vi "Master Save.vi"(7 "#scans":u32, 8 "Current Scan #":u32, 10 "Data Store":T1, 11 "File IO in":refnum<class "File IO.lvclass">) -> (0 "error out":errorcluster, 3 "File IO out":refnum<class "File IO.lvclass">)   [LabVIEW 2012, in "File IO.lvclass"]
uses:
  File IO.lvclass
  Instruments/Utility Classes/Readable/Data Store.ctl
  Instruments/Utility Classes/Readable/Data Point.ctl
  Instruments/Utility Classes/Readable/Time.ctl
  Instruments/Utility Classes/Readable/X.ctl
  File IO.lvclass/File IO.ctl
  <vilib>/Utility/file.llb/Write To Spreadsheet File (DBL).vi
  Data File Header Constants.vi
  Instruments/Utility Classes/Readable/Readable.lvclass
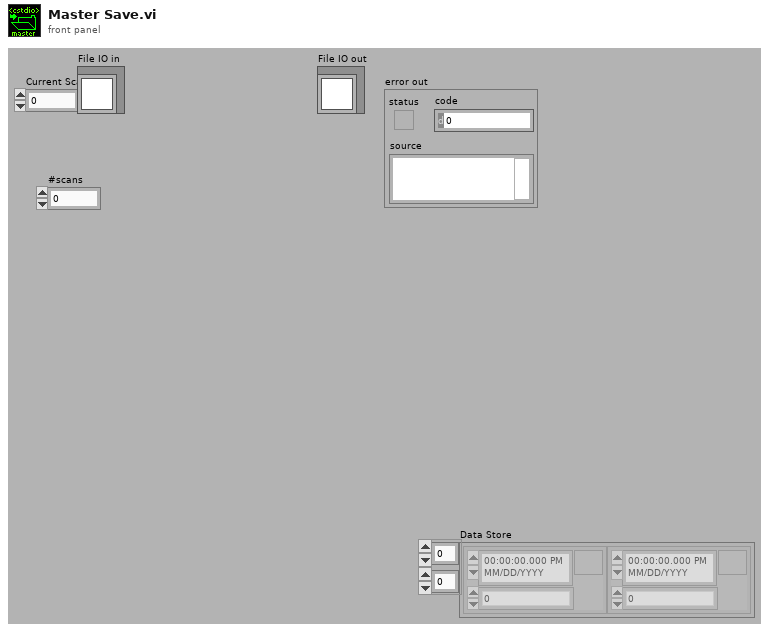
[diagram p1: front panel]
types:
  T1 = typedef "Readable.lvclass/Data Store.ctl" = T2[][]
  T2 = typedef "Readable.lvclass/Data Point.ctl" = cluster{"t":T3, "x":T4}
  T3 = typedef "Readable.lvclass/Time.ctl" = timestamp
  T4 = typedef "Readable.lvclass/X.ctl" = dbl
  T5 = enum16{"open", "replace", "create", "open or create", "replace or create", "replace or create with confirmation"}
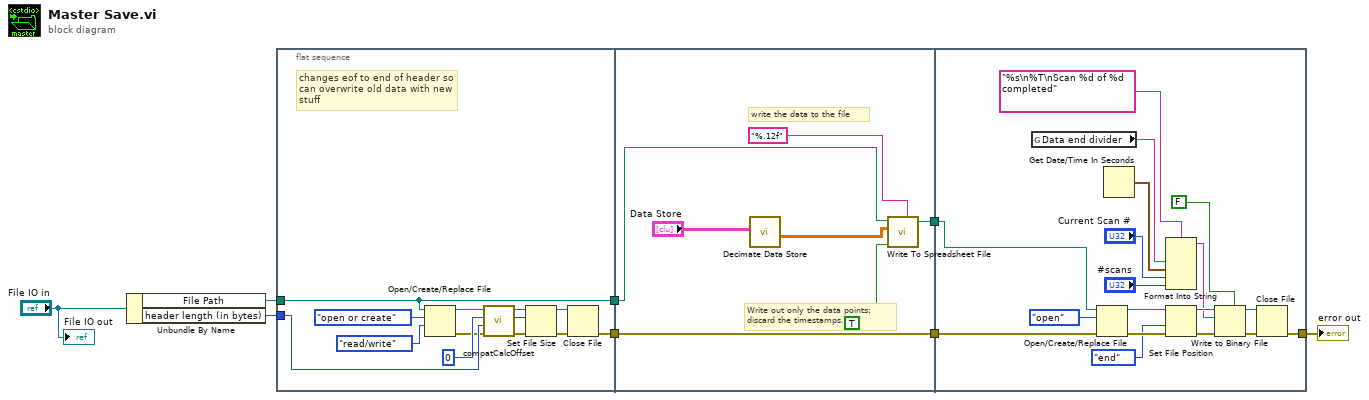
[diagram p0: block diagram]
diagram:
  n1 = Unbundle By Name("File IO in") -> ("File Path"=w7:path, "header length (in bytes)"=w4:u64)
  n2 = flat-sequence {
    tunnel: w7 -> [w13]
    tunnel: [w13] -> w6
    tunnel: w4 -> [w12]
    tunnel: [w9] -> w2
    tunnel: w6 -> [w25]
    tunnel: [w24] -> w5
    tunnel: [w26] -> w3
    tunnel: w2 -> [w26]
    tunnel: w5 -> [w33]
    tunnel: w3 -> [w32]
    tunnel: [w30] -> w1
    frame #0 {
      # "changes eof to end of header so\ncan overwrite old data with new\nstuff"
      n3 = Open/Create/Replace File(file path (use dialog)=w13, operation (0:open)=T5."open or create", access (0:read/write)=enum16{"read/write", "read-only", "write-only"}."read/write") -> (refnum out=w14:refnum<file>, error out=w11:errorcluster)  [unwired: 1 in, 3 out]
      n4 = call <vilib>:"compatCalcOffset.vi"("error in"=w11, "pos offset (0)"=w12, "pos mode (0:1)"=u16 0, "refnum"=w14) -> ("error out"=w20:errorcluster, "offset"=w19:i32, "dup refnum"=w18:refnum<file>)  [unwired: 5 out]
      n5 = Set File Size(4:w20, 6:w19, 7:w18) -> (0:w10:errorcluster, 3:w17:refnum<file>)
      n6 = Close File(refnum=w17, error in=w10) -> (error out=w9:errorcluster)  [unwired: 1 out]
    }
    frame #1 {
      # "Write out only the data points;\ndiscard the timestamps."
      # "write the data to the file"
      n7 = call "Decimate Data Store.vi"("Data Store"="Data Store") -> ("Data Points"=w22:T4[][])  [unwired: 9 in, 1 out]
      n8 = call-poly <vilib>:"Write To Spreadsheet File.vi"("format (%.3f)"="%.12f", "append to file? (new file:F)"=TRUE, "2D data"=w22, "file path (dialog if empty)"=w25) -> ("new file path (Not A Path if cancelled)"=w24:path)  [unwired: 2 in, 2 out]
    }
    frame #2 {
      n9 = global read "Data File Header Constants.vi" "Data end divider"() -> (w39:string)
      n10 = Open/Create/Replace File(file path (use dialog)=w33, error in=w32, operation (0:open)=T5."open") -> (refnum out=w44:refnum<file>, error out=w42:errorcluster)  [unwired: 1 in, 3 out]
      n11 = Get Date/Time In Seconds() -> (seconds since 1Jan1904=w38:timestamp)
      n12 = Format Into String(format string="%s\n%T\nScan %d of %d completed", w39, w38, "Current Scan #", "#scans") -> (resulting string=w37:string)  [unwired: 2 in, 1 out]
      n13 = Set File Position(refnum=w44, from (0:start)=enum16{"start", "end", "current"}."end", error in=w42) -> (refnum out=w45:refnum<file>, error out=w46:errorcluster)  [unwired: 1 out]
      n14 = Write to Binary File(file (use dialog)=w45, data=w37, error in=w46, 5:FALSE ("prepend array or string size? (T)")) -> (refnum out=w43:refnum<file>, error out=w31:errorcluster)  [unwired: 3 out]
      n15 = Close File(refnum=w43, error in=w31) -> (error out=w30:errorcluster)  [unwired: 1 out]
    }
  }
  "File IO out" <- "File IO in"
  "error out" <- w1
